vi "imaq set timeout.vi"(8 "error in (no error)":errorcluster, 10 "timeout":dbl, 11 "Point Grey Camera in":refnum<class "Point Grey Camera.lvclass">) -> (0 "error out":errorcluster, 3 "FakeCamera out":refnum<class "Point Grey Camera.lvclass">)   [LabVIEW 2020, in "Point Grey Camera.lvclass"]
uses:
  Point Grey Camera.lvclass
  <resource>/objmgr/imaqdx.rc
  <vilib>/vision/driver/NI_Vision_Acquisition_Software.lvlib
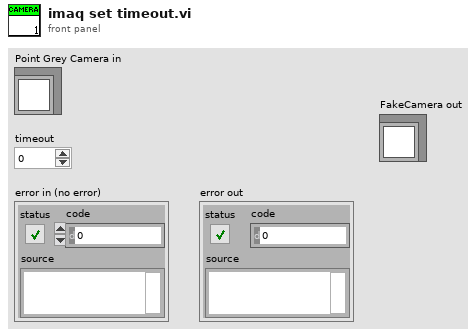
[diagram p1: front panel]
types:
  T1 = typedef "IMAQdx.ctl" = refnum<k21>
  T2 = typedef "OnOffTypeDef.ctl" = enum16{"off", "on"}
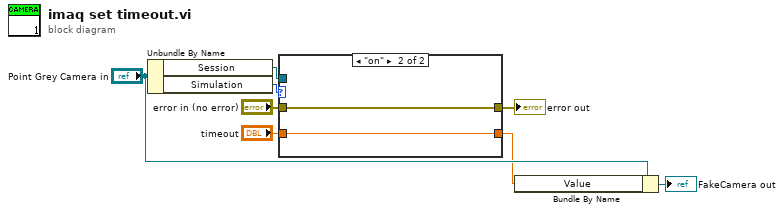
[diagram p0: block diagram]
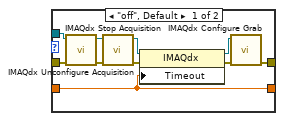
[diagram p2: hidden frame]
diagram:
  n1 = Unbundle By Name("Point Grey Camera in") -> ("Session"=w6:T1, "Simulation"=w2:T2)
  n2 = case shown="\"on\"" w2 {
    tunnel: [w18 w20] -> w8
    tunnel: "error in (no error)" -> [w16 w20]
    tunnel: w6 -> [w11 _]
    tunnel: "timeout" -> [w9 w19]
    tunnel: [w9 w19] -> w1
    frame "off", Default {
      n3 = call <vilib>:"IMAQdx Stop Acquisition.vi"("error in"=w16, "Session In"=w11) -> ("error out"=w14:errorcluster, "Session Out"=w10:T1)  [unwired: 8 out]
      n4 = call <vilib>:"IMAQdx Unconfigure Acquisition.vi"("error in"=w14, "Session In"=w10) -> ("error out"=w15:errorcluster, "Session Out"=w12:T1)  [unwired: 8 out]
      n5 = property class="IMAQdx"(reference=w12, error in=w15, "Timeout"=w9) -> (reference out=w13:T1, error out=w17:errorcluster)
      n6 = call <vilib>:"IMAQdx Configure Grab.vi"("error in"=w17, "Session In"=w13) -> ("error out"=w18:errorcluster)  [unwired: 1 in, 8 out]
    }
    frame "on" {
    }
  }
  "error out" <- w8
  n7 = Bundle By Name(cluster="Point Grey Camera in", "Value"=w1) -> (→"FakeCamera out":refnum<class "Point Grey Camera.lvclass">)
